vi "stackErrorSimple.vi"(10 "Second Error In":u32, 11 "First Error In":u32) -> (3 "Error Out":u32)   [LabVIEW 2017]
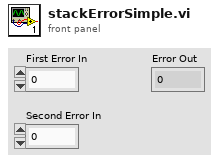
[diagram p1: front panel]
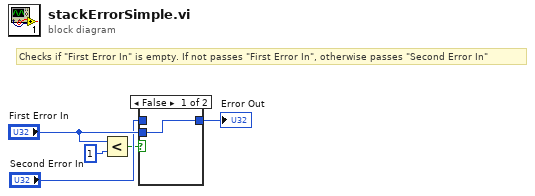
[diagram p0: block diagram]
diagram:
  # "Checks if \"First Error In\" is empty. If not passes \"First Error In\", otherwise passes \"Second Error In\""
  n1 = Less?(x="First Error In", y=1) -> (x < y?=w2:bool)
  n2 = case shown="False" w2 {
    tunnel: "Second Error In" -> [_ w7]
    tunnel: [w6 w7] -> w4
    tunnel: "First Error In" -> [w6 _]
    frame False {
    }
    frame True {
    }
  }
  "Error Out" <- w4
